vi "DrawGbox.vi"(1 "Object in":refnum<vi>, 3 "Color":T1={"Red"=0.0, "Green"=1.0, "Blue"=0.0, "Alpha"=1.0}, 4 "contents":string) -> (0 "Object out":refnum<vi>, 2 "remaining":string)   [LabVIEW 2010]
uses:
  <vilib>/picture/3D Picture Control/NI_3D Picture Control.lvlib
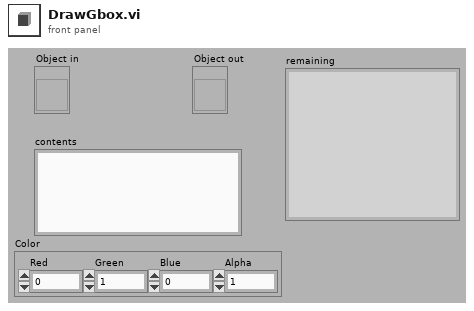
[diagram p1: front panel]
types:
  T1 = cluster{"Red":sgl, "Green":sgl, "Blue":sgl, "Alpha":sgl}
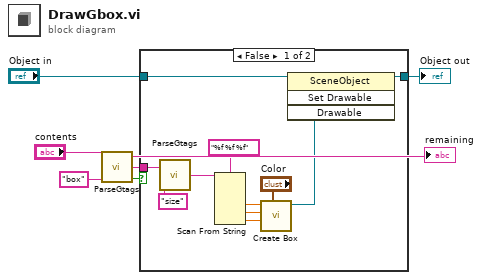
[diagram p0: block diagram]
diagram:
  n1 = call "ParseGtags.vi"("tag"="box", "urdf in"="contents") -> ("not found"=w4:bool, "contents"=w5:string, "urdf out"=→"remaining":string)  [unwired: 1 out]
  n2 = case shown="False" w4 {
    tunnel: w5 -> [w17 _]
    tunnel: "Object in" -> [w15 w19]
    tunnel: [w14 w19] -> w7
    frame False {
      n3 = call "ParseGtags.vi"("tag"="size", "urdf in"=w17) -> ("contents"=w16:string)  [unwired: 3 out]
      n4 = Scan From String(format string="%f %f %f", input string=w16) -> (output 1=w12:dbl, output 2=w11:dbl, output 3=w10:dbl)  [unwired: 5 in, 3 out]
      n5 = call <vilib>:"Create Box.vi"("Color"="Color", "Length Z"=w10, "Length Y"=w11, "Length X"=w12) -> ("New Box Refnum"=w9:refnum<vi>)  [unwired: 6 in, 1 out]
      n6 = invoke class="SceneObject" method="Set Drawable"(reference=w15, "Drawable"=w9) -> (reference out=w14:refnum<vi>)  [unwired: 2 in, 3 out]
    }
    frame True {
    }
  }
  "Object out" <- w7
